vi "ReadExpectedDependencies.vi"(8 "error in (no error)":errorcluster, 11 "Library/Class Path":path) -> (0 "error out":errorcluster, 1 "ExpectedDeps Path":path, 2 "Expected Indirect Dependencies":string[](array[string]), 3 "Expected Direct Dependencies":string[](array[string]), 5 "Found?":bool)   [LabVIEW 2019, in "Hawkeye.lvlib"]
uses:
  Hawkeye.lvlib
  <vilib>/Utility/config.llb/NI_LVConfig.lvlib
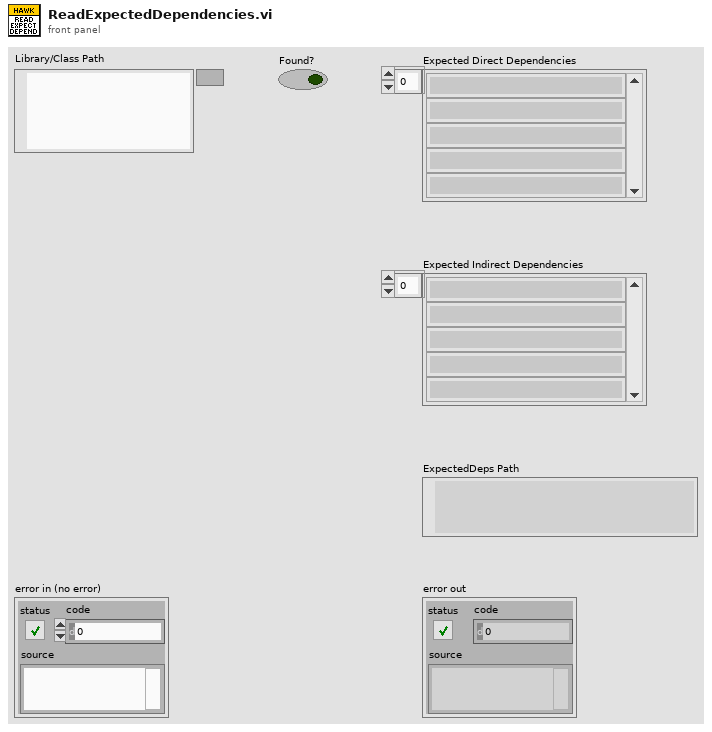
[diagram p1: front panel]
types:
  T1 = typedef "NI_LVConfig.lvlib/Config Data RefNum.ctl" = refnum<k1>
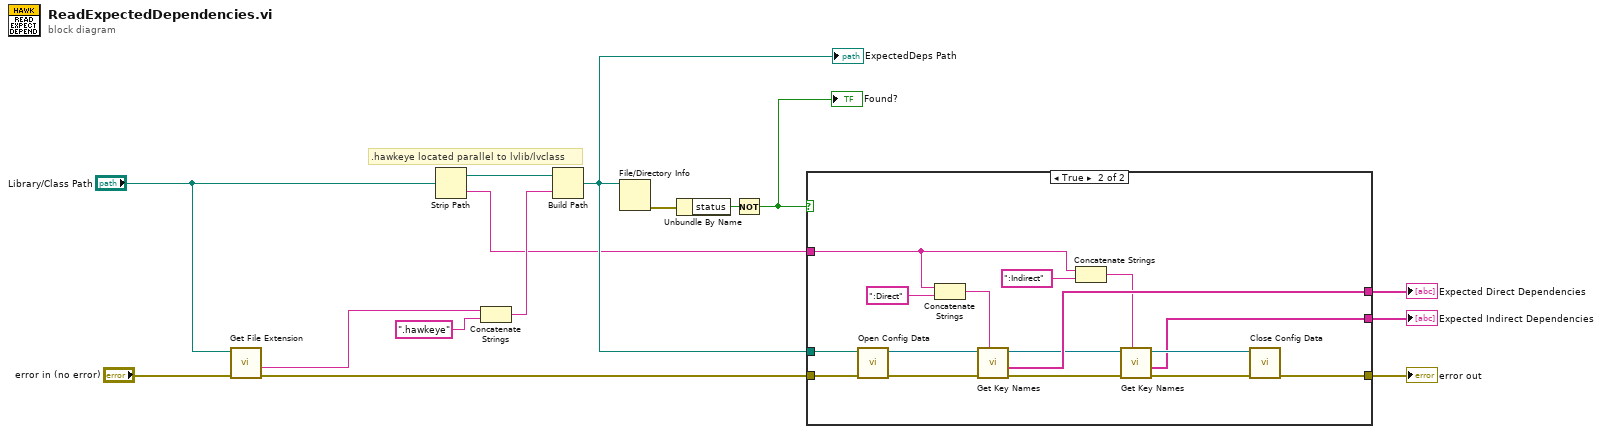
[diagram p0: block diagram]
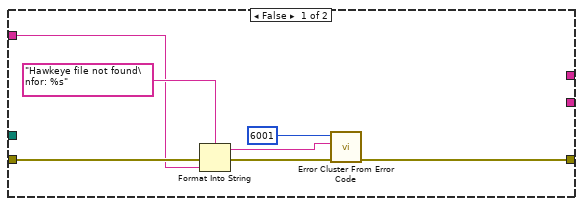
[diagram p2: hidden frame]
diagram:
  # ".hawkeye located parallel to lvlib/lvclass"
  n1 = call <vilib>:"Get File Extension.vi"("error in (no error)"="error in (no error)", "file"="Library/Class Path") -> ("error out"=w4:errorcluster, "filename without extension"=w3:string)  [unwired: 5 in, 3 out]
  n2 = Strip Path(path="Library/Class Path") -> (stripped path=w15:path, name=w2:string)
  n3 = Concatenate Strings(w3, ".hawkeye" ("string")) -> (w13:string)
  n4 = Build Path(base path=w15, name or relative path=w13) -> (appended path=w10:path)
  "ExpectedDeps Path" <- w10
  n5 = File/Directory Info(path=w10) -> (error out=w7:errorcluster)  [unwired: 1 in, 6 out]
  n6 = Unbundle By Name(w7) -> ("status"=w8:bool)
  n7 = Not(x=w8) -> (.not. x?=w9:bool)
  "Found?" <- w9
  n8 = case shown="True" w9 {
    tunnel: w4 -> [w21 w38]
    tunnel: w2 -> [w19 w23]
    tunnel: [w16 w33] -> w12
    tunnel: w10 -> [_ w37]
    tunnel: [_ w34] -> w11
    tunnel: [_ w25] -> w6
    frame False {
      n9 = Format Into String(format string="Hawkeye file not found\nfor: %s" ("error message (\"\")"), error in=w21, w19) -> (resulting string=w18:string, error out=w17:errorcluster)  [unwired: 1 in]
      n10 = call <vilib>:"Error Cluster From Error Code.vi"("error in (no error)"=w17, "error message (\"\")"=w18, "error code (0)"=6001) -> ("error out"=w16:errorcluster)  [unwired: 6 in]
    }
    frame True {
      n11 = call <vilib>:"Open Config Data.vi"("error in (no error)"=w38, "configuration file path"=w37) -> ("error out"=w36:errorcluster, "refnum"=w35:T1)  [unwired: 7 in, 1 out]
      n12 = Concatenate Strings(w23, ":Direct" ("string")) -> (w24:string)
      n13 = call <vilib>:"Get Key Names.vi"("section"=w24, "error in (no error)"=w36, "refnum"=w35) -> ("error out"=w28:errorcluster, "key names"=w34:string[], "refnum out"=w30:T1)  [unwired: 5 in, 1 out]
      n14 = Concatenate Strings(w23, ":Indirect" ("string")) -> (w26:string)
      n15 = call <vilib>:"Get Key Names.vi"("section"=w26, "error in (no error)"=w28, "refnum"=w30) -> ("error out"=w27:errorcluster, "key names"=w25:string[], "refnum out"=w29:T1)  [unwired: 5 in, 1 out]
      n16 = call <vilib>:"Close Config Data.vi"("error in (no error)"=w27, "refnum"=w29) -> ("error out"=w33:errorcluster)  [unwired: 8 in, 1 out]
    }
  }
  "error out" <- w12
  "Expected Direct Dependencies" <- w11
  "Expected Indirect Dependencies" <- w6
